vi "PRIME Copy Raw Files.vi"(8 "error in":errorcluster, 9 "Source Files":path[](array[path]), 10 "Filenames":string[](array[string])=["0001C1.fits", "0001C2.fits", "0001C3.fits", "0001C4.fits", "0002C1.fits", "0002C2.fits", "0002C3.fits", "0002C4.fits", "0003C1.fits", "0003C2.fits", "0003C3.fits", "0003C4.fits", "0004C1.fits", "0004C2.fits", "0004C3.fits", "0004C4.fits", "0005C1.fits", "0005C2.fits", "0005C3.fits", "0005C4.fits", "0006C1.fits", "0006C2.fits", "0006C3.fits", "0006C4.fits", "0007C1.fits", "0007C2.fits", "0007C3.fits", "0007C4.fits", "0008C1.fits", "0008C2.fits", "0008C3.fits", "0008C4.fits"], 11 "target path":path) -> (0 "error out":errorcluster, 2 "files":path[](array[path]), 3 "This Acq Image Folder":path)   [LabVIEW 2024, in "PRIME Detector.lvclass"]
uses:
  PRIME Detector.lvclass
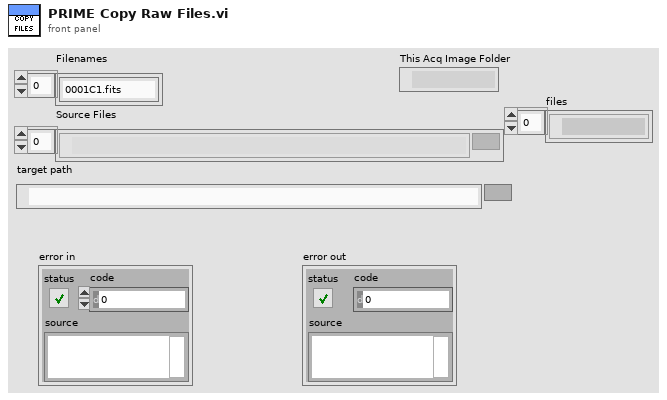
[diagram p1: front panel]
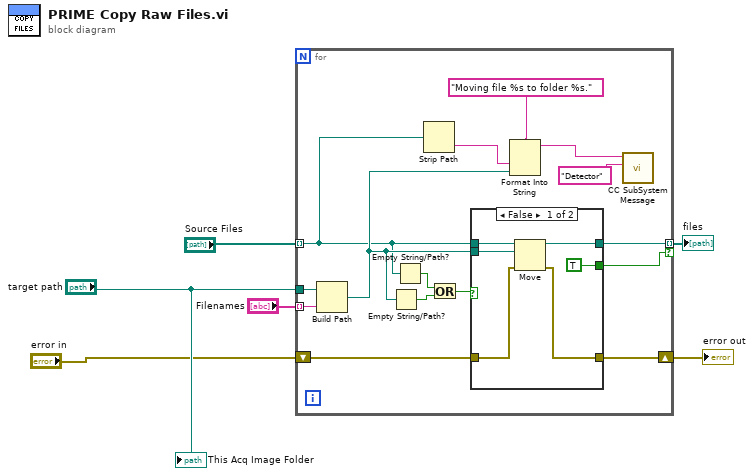
[diagram p0: block diagram]
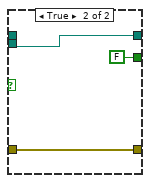
[diagram p2: hidden frame]
diagram:
  n1 = for {
    tunnel: "Source Files" -> [w11] mode=indexing
    tunnel: "Filenames" -> [w21] mode=indexing
    tunnel: "target path" -> [w20]
    shift-right: [w18] -> w4
    shift-left: "error in" -> [w19]
    tunnel: [w13] -> w1 mode=indexing if=w7
    n2 = Build Path(base path=w20, name or relative path=w21) -> (appended path=w12:path)
    n3 = Empty String/Path?(string/path=w12) -> (empty?=w9:bool)
    n4 = Empty String/Path?(string/path=w11) -> (empty?=w8:bool)
    n5 = Strip Path(path=w11) -> (name=w16:string)  [unwired: 1 out]
    n6 = Or(x=w8, y=w9) -> (x .or. y?=w10:bool)
    n7 = case shown="False" w10 {
      tunnel: w19 -> [w27 w29]
      tunnel: [w26 w29] -> w18
      tunnel: [w25 w30] -> w13
      tunnel: w12 -> [w24 w30]
      tunnel: w11 -> [w23 _]
      tunnel: [TRUE FALSE] -> w7
      frame False {
        n8 = Move(source path=w23, error in=w27, 10:w24) -> (error out=w26:errorcluster, 3:w25:path)  [unwired: 2 in, 1 out]
      }
      frame True {
      }
    }
    n9 = Format Into String(format string="Moving file %s to folder %s.", w16, w12) -> (resulting string=w14:string)  [unwired: 2 in, 1 out]
    n10 = call "CC SubSystem Message.vi"("Subsystem"="Detector", "Message"=w14) -> ()  [unwired: 9 in, 1 out]
  }
  "error out" <- w4
  "files" <- w1
  "This Acq Image Folder" <- "target path"
